vi "Fiinal Block Diagram.vi"() -> ()   [LabVIEW 2017]
panel:
  in  "?":dbl=1.0 min=1.0 max=10.0 step=1.0
  in  "?":dbl=1.0 min=1.0 max=10.0 step=1.0
  in  "?":dbl=1.0 min=1.0 max=10.0 step=1.0
  in  "?":dbl=1.0 min=1.0 max=10.0 step=1.0
  in  "Quantity":dbl=1.0 min=1.0 max=10.0 step=1.0
  out "Your Order Will Be Prepared In":dbl
  in  "Pay Bill and Confirm":bool
  out "Discount":string
  out "Total Bill":dbl
  out "?":dbl
  in  "Poha":bool
  out "?":dbl
  in  "Idli":bool
  out "?":dbl
  in  "Dosa":bool
  out "?":dbl
  in  "Noodles":bool
  out "Price":dbl
  in  "Chocolate Shake":bool
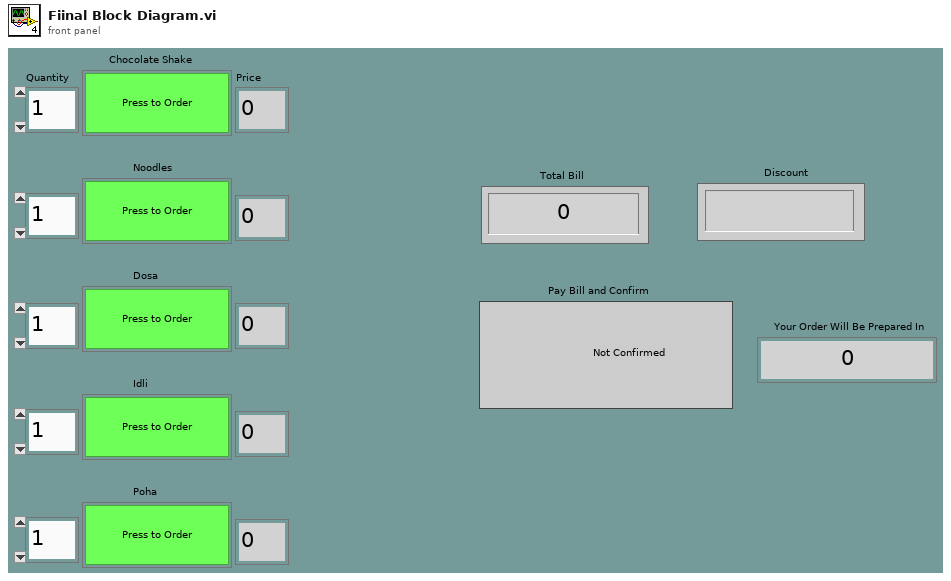
[diagram p1: front panel]
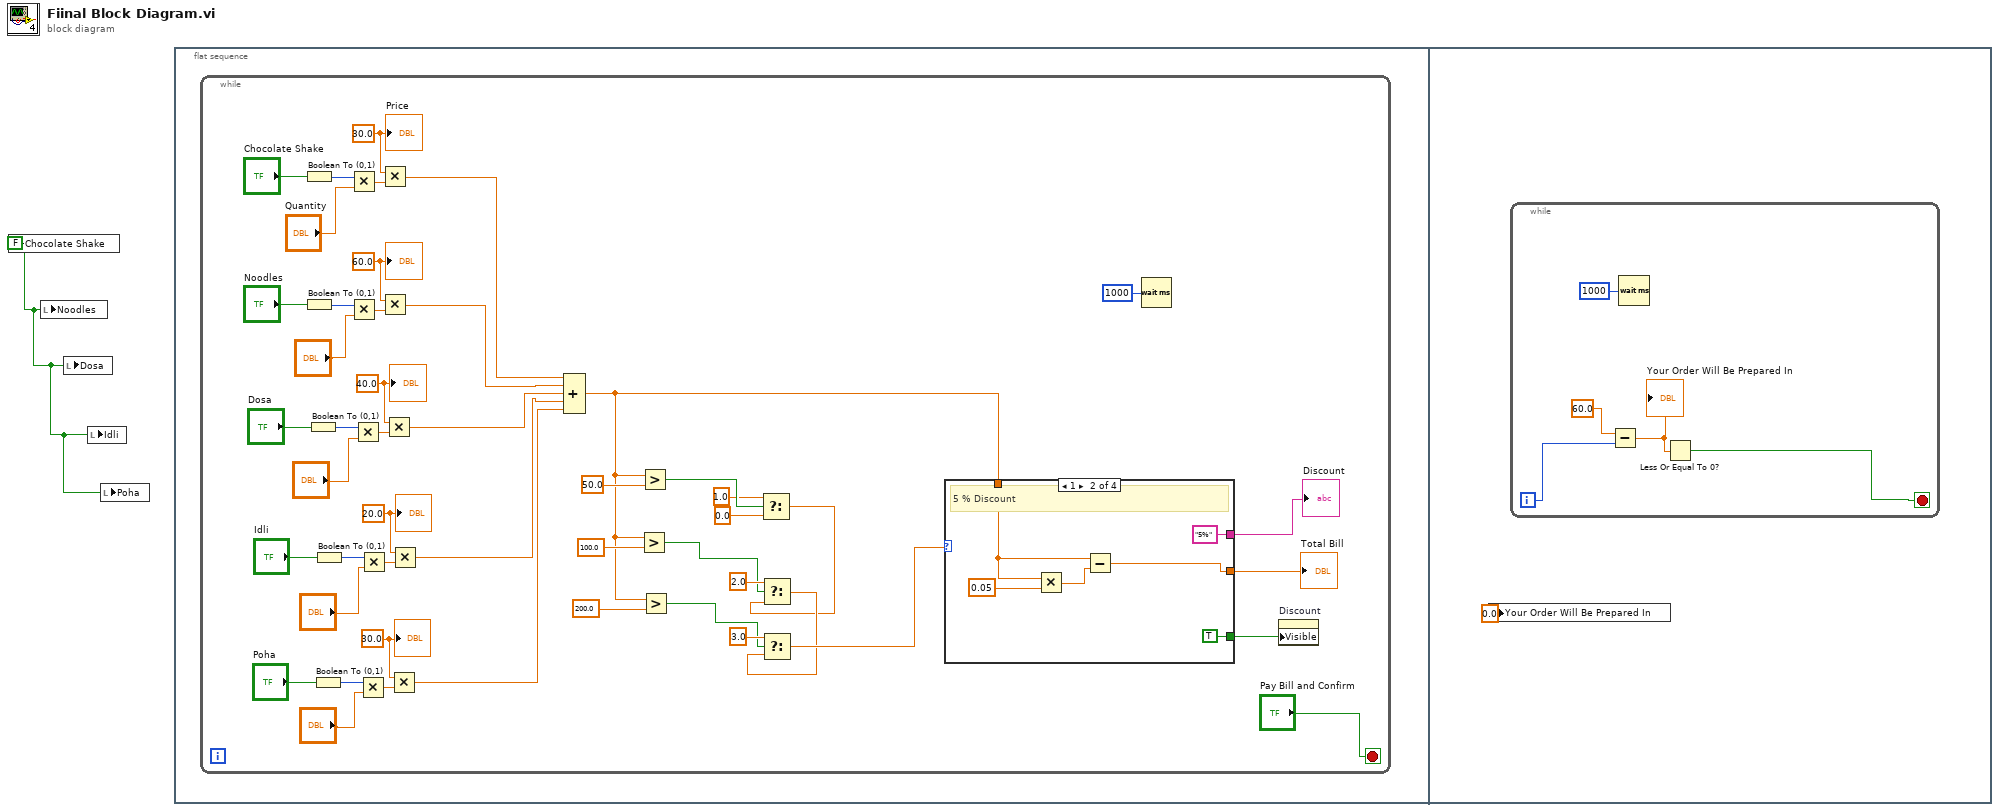
[diagram p0: block diagram]
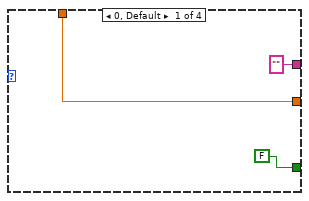
[diagram p2: hidden frame]
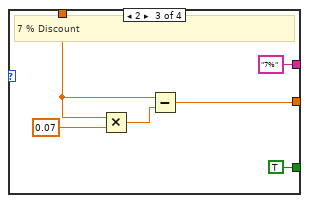
[diagram p3: hidden frame]
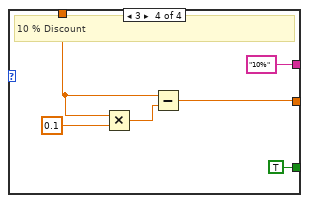
[diagram p4: hidden frame]
diagram:
  w1 = FALSE ("Item # 1")
  n1 = local write "Chocolate Shake"(w1) -> ()
  n2 = local write "Noodles"(w1) -> ()
  n3 = local write "Dosa"(w1) -> ()
  n4 = local write "Idli"(w1) -> ()
  n5 = local write "Poha"(w1) -> ()
  n6 = flat-sequence {
    frame #0 {
      n7 = while {
        stop <- "Pay Bill and Confirm" stop-if-true
        w31 = 30.0 ("Price")
        w35 = 20.0 ("Price")
        w39 = 40.0 ("Price")
        w43 = 60.0 ("Price")
        w47 = 30.0 ("Price")
        n8 = Boolean To (0,1)(Boolean="Chocolate Shake") -> (0, 1=w49:i16)
        n9 = Boolean To (0,1)(Boolean="Noodles") -> (0, 1=w45:i16)
        n10 = Boolean To (0,1)(Boolean="Dosa") -> (0, 1=w41:i16)
        n11 = Boolean To (0,1)(Boolean="Poha") -> (0, 1=w33:i16)
        n12 = Boolean To (0,1)(Boolean="Idli") -> (0, 1=w37:i16)
        n13 = Multiply(x=w49, y="Quantity") -> (x*y=w48:dbl)
        n14 = Multiply(x=w45, y="?") -> (x*y=w44:dbl)
        n15 = Multiply(x=w41, y="?") -> (x*y=w40:dbl)
        n16 = Multiply(x=w33, y="?") -> (x*y=w32:dbl)
        n17 = Multiply(x=w37, y="?") -> (x*y=w36:dbl)
        n18 = Multiply(x=w47, y=w48) -> (x*y=w30:dbl)
        n19 = Multiply(x=w43, y=w44) -> (x*y=w29:dbl)
        n20 = Multiply(x=w39, y=w40) -> (x*y=w28:dbl)
        n21 = Multiply(x=w31, y=w32) -> (x*y=w26:dbl)
        n22 = Multiply(x=w35, y=w36) -> (x*y=w27:dbl)
        n23 = Compound Arithmetic op=ADD(w30, w29, w28, w27, w26) -> (w17:dbl)
        n24 = Greater?(x=w17, y=100.0) -> (0:w13:bool)
        n25 = Greater?(x=w17, y=50.0) -> (0:w11:bool)
        n26 = Greater?(x=w17, y=200.0) -> (0:w20:bool)
        n27 = Select(t=1.0, s=w11, f=0.0) -> (s? t:f=w8:dbl)
        n28 = Select(t=2.0, s=w13, f=w8) -> (s? t:f=w12:dbl)
        n29 = Select(t=3.0, s=w20, f=w12) -> (s? t:f=w18:dbl)
        n30 = case shown="1" w18 {
          tunnel: [w53 w56 w62 w68] -> w19
          tunnel: w17 -> [w53 w57 w63 w69]
          tunnel: ["" ("Discount") "5%" ("Discount") "7%" ("Discount") "10%" ("Discount")] -> w16
          tunnel: [FALSE ("Visible") TRUE ("Visible") TRUE ("Visible") TRUE ("Visible")] -> w7
          frame 0, Default {
          }
          frame 1 {
            # "5 % Discount"
            n31 = Multiply(x=w57, y=0.05) -> (x*y=w58:dbl)
            n32 = Subtract(x=w57, y=w58) -> (x-y=w56:dbl)
          }
          frame 2 {
            # "7 % Discount"
            n33 = Multiply(x=w63, y=0.07) -> (x*y=w65:dbl)
            n34 = Subtract(x=w63, y=w65) -> (x-y=w62:dbl)
          }
          frame 3 {
            # "10 % Discount"
            n35 = Multiply(x=w69, y=0.1) -> (x*y=w71:dbl)
            n36 = Subtract(x=w69, y=w71) -> (x-y=w68:dbl)
          }
        }
        "Total Bill" <- w19
        "Discount" <- w16
        n37 = Wait (ms)(milliseconds to wait=u32 1000) -> ()  [unwired: 1 out]
        n38 = property on="Discount" class="Str"("Visible"=w7) -> ()  [unwired: 2 in, 2 out]
        "Price" <- w47
        "?" <- w43
        "?" <- w39
        "?" <- w35
        "?" <- w31
      }
    }
    frame #1 {
      n39 = local write "Your Order Will Be Prepared In"(0.0 ("Your Order Will Be Prepared In")) -> ()
      n40 = while {
        i -> [w76]
        stop <- w74 stop-if-true
        n41 = Subtract(x=60.0, y=w76) -> (x-y=w75:dbl)
        "Your Order Will Be Prepared In" <- w75
        n42 = Wait (ms)(milliseconds to wait=u32 1000) -> ()  [unwired: 1 out]
        n43 = Less Or Equal To 0?(x=w75) -> (x <= 0?=w74:bool)
      }
    }
  }
